vi "FringeTrackerOpenSynchronization.vi"(9 "error in (no error)":errorcluster) -> (2 "FringeTrackerSynchro":T1, 6 "error out":errorcluster)   [LabVIEW 2009]
uses:
  Controls/FringeTrackerSynchro.ctl
  Controls/FringTrackerCommand.ctl
  Controls/FringeTrackerData.ctl
  Nicmos/Controls/NICMOS.READOUT.ctl
  Controls/FringeTrackerState.ctl
  Controls/FringeTrackerInfo.ctl
  Nicmos/Controls/NICMOS.DATA.ctl
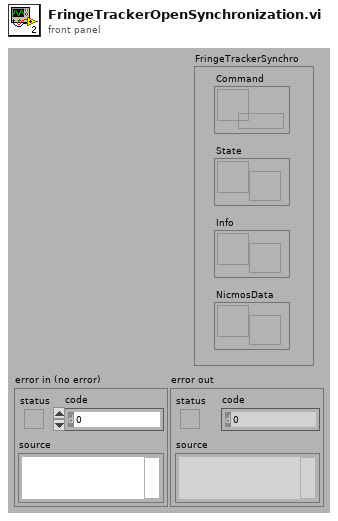
[diagram p1: front panel]
types:
  T1 = typedef "FringeTrackerSynchro.ctl" = cluster{"Command":refnum<queue>, "State":refnum<notifier>, "Info":refnum<notifier>, "NicmosData":refnum<notifier>}
  T2 = typedef "NICMOS.DATA.ctl" = cluster{"DATA":i32[][][], "INDEX":i32}
  T3 = typedef "FringeTrackerInfo.ctl" = cluster{"Readout":T4, "OPD stroke":dbl[unit], "OPD per pixel":dbl[unit]}
  T4 = typedef "NICMOS.READOUT.ctl" = cluster{"Readout":i32, "Deglitch":i32, "Framerate":dbl[unit], "Bank":i32}
  T5 = typedef "FringeTrackerState.ctl" = enum16{"IDLING", "CONFIGURING", "SCANNING", "SEARCHING", "TRACKING", "STOPPING"}
  T6 = typedef "FringTrackerCommand.ctl" = cluster{"Command":enum16{"IDLE", "SCAN", "TRACK", "QUIT"}, "FringeTrackerData":T7}
  T7 = typedef "FringeTrackerData.ctl" = cluster{"Readout":T4, "Wavelength":dbl[unit], "Frame per fringe":dbl, "Autcollimation":bool, "OPD stroke":dbl[unit], "OPD per pixel":dbl[unit], "Offset":dbl[unit]}
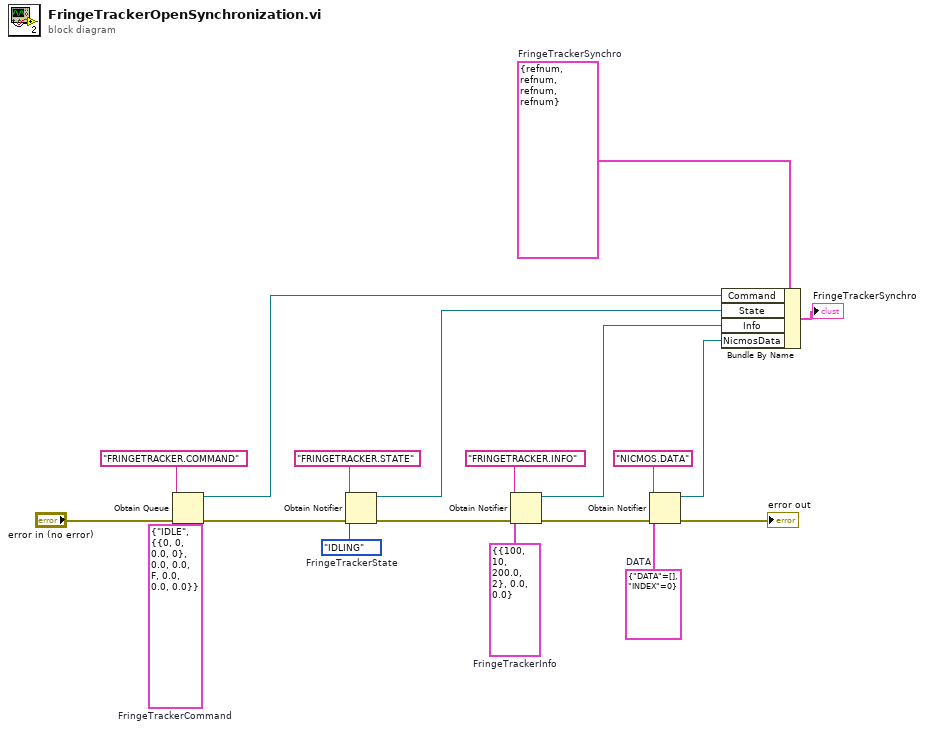
[diagram p0: block diagram]
diagram:
  w3 = T2 {"DATA"=[], "INDEX"=0}  # DATA
  w7 = T3 {"Readout"={"Readout"=100, "Deglitch"=10, "Framerate"=200.0, "Bank"=2}, "OPD stroke"=0.0, "OPD per pixel"=0.0}  # FringeTrackerInfo
  w13 = T1 {"Command"=refnum, "State"=refnum, "Info"=refnum, "NicmosData"=refnum}  # FringeTrackerSynchro
  w14 = FringeTrackerState."IDLING"  # FringeTrackerState
  w9 = T6 {"Command"=enum."IDLE", "FringeTrackerData"={"Readout"={"Readout"=0, "Deglitch"=0, "Framerate"=0.0, "Bank"=0}, "Wavelength"=0.0, "Frame per fringe"=0.0, "Autcollimation"=FALSE, "OPD stroke"=0.0, "OPD per pixel"=0.0, "Offset"=0.0}}  # FringeTrackerCommand
  n1 = Obtain Queue(name (unnamed)="FRINGETRACKER.COMMAND", element data type=w9, error in (no error)="error in (no error)") -> (queue out=w12:refnum<queue>, error out=w16:errorcluster)  [unwired: 2 in, 1 out]
  n2 = Obtain Notifier(name (unnamed)="FRINGETRACKER.STATE", notification data type=w14, error in (no error)=w16) -> (notifier out=w11:refnum<notifier>, error out=w5:errorcluster)  [unwired: 1 in, 1 out]
  n3 = Obtain Notifier(name (unnamed)="FRINGETRACKER.INFO", notification data type=w7) -> (notifier out=w6:refnum<notifier>)  [unwired: 2 in, 2 out]
  n4 = Obtain Notifier(name (unnamed)="NICMOS.DATA", notification data type=w3, error in (no error)=w5) -> (notifier out=w1:refnum<notifier>, error out=→"error out":errorcluster)  [unwired: 1 in, 1 out]
  n5 = Bundle By Name(cluster=w13, "Command"=w12, "State"=w11, "Info"=w6, "NicmosData"=w1) -> (→"FringeTrackerSynchro":T1)
